vi "VerifPreDCIR.vi"(8 "errin":errorcluster, 11 "VISA resource name":refnum<visa-resource-name>) -> (0 "errout":errorcluster caption="sortie d'erreur", 3 "V>35 ?":bool)   [LabVIEW 2020]
uses:
  5f35586e-bf77-4ad9-b645-b9e33e4f06e5.vi
  <instrlib>/IT6000C/IT6000C.lvlib
panel:
  out "Actual Voltage Level (V)":dbl format="%.2g"
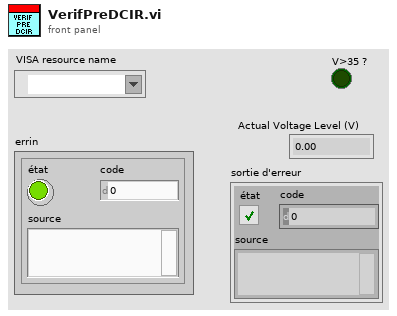
[diagram p1: front panel]
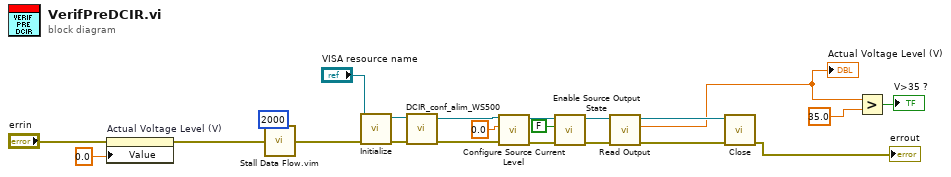
[diagram p0: block diagram]
diagram:
  n1 = property on="Actual Voltage Level (V)" class="DigNum (strict)"(error in="errin", "Value"=0.0 ("Actual Voltage Level (V)")) -> (error out=w5:errorcluster)  [unwired: 1 in, 1 out]
  n2 = call "Stall Data Flow.vim"("value in"=w5, "milliseconds to wait"=u32 2000) -> ("value out"=w9:errorcluster)  [unwired: 1 out]
  n3 = call <instrlib>:"Initialize.vi"("error in (no error)"=w9, "VISA resource name"="VISA resource name") -> ("error out"=w8:errorcluster, "VISA resource name out"=w10:refnum<visa-resource-name>)  [unwired: 8 in]
  n4 = call "DCIR_conf_alim_WS500.vi"("ErrIN"=w8, "VISAin"=w10) -> ("ErrOUT"=w21:errorcluster, "VisaOUT"=w20:refnum<visa-resource-name>)  [unwired: 8 in]
  n5 = call <instrlib>:"Configure Source Current Level.vi"("error in (no error)"=w21, "Value(0)"=0.0, "VISA resource name"=w20) -> ("error out"=w19:errorcluster, "VISA resource name out"=w18:refnum<visa-resource-name>)  [unwired: 7 in]
  n6 = call <instrlib>:"Enable Source Output State.vi"("error in (no error)"=w19, "Enable(True)"=FALSE, "VISA resource name"=w18) -> ("error out"=w15:errorcluster, "VISA resource name out"=w14:refnum<visa-resource-name>)  [unwired: 7 in]
  n7 = call <instrlib>:"Read Output.vi"("error in (no error)"=w15, "VISA resource name"=w14) -> ("error out"=w13:errorcluster, "Actual Voltage Level (V)"=w4:dbl, "VISA resource name out"=w12:refnum<visa-resource-name>)  [unwired: 6 in, 1 out]
  "Actual Voltage Level (V)" <- w4
  n8 = call <instrlib>:"Close.vi"("error in (no error)"=w13, "VISA resource name"=w12) -> ("error out"=→"errout":errorcluster)  [unwired: 9 in]
  n9 = Greater?(x=w4, y=35.0) -> (0:→"V>35 ?":bool)
